vi "AddValue.vi"(1 "Display State In":T2 caption="State", 2 "Data In":T1) -> (0 "Display State Out":T2 caption="State")   [LabVIEW 2013, in "VariantXControl__VP.xctl"]
uses:
  VariantXControl__VP.xctl
  VariantState.ctl
  Permissions.ctl
  TreeSettings.ctl
  VariantData.ctl
  VariantTree__VP.lvclass
  Browse Variant_SetRef.vi
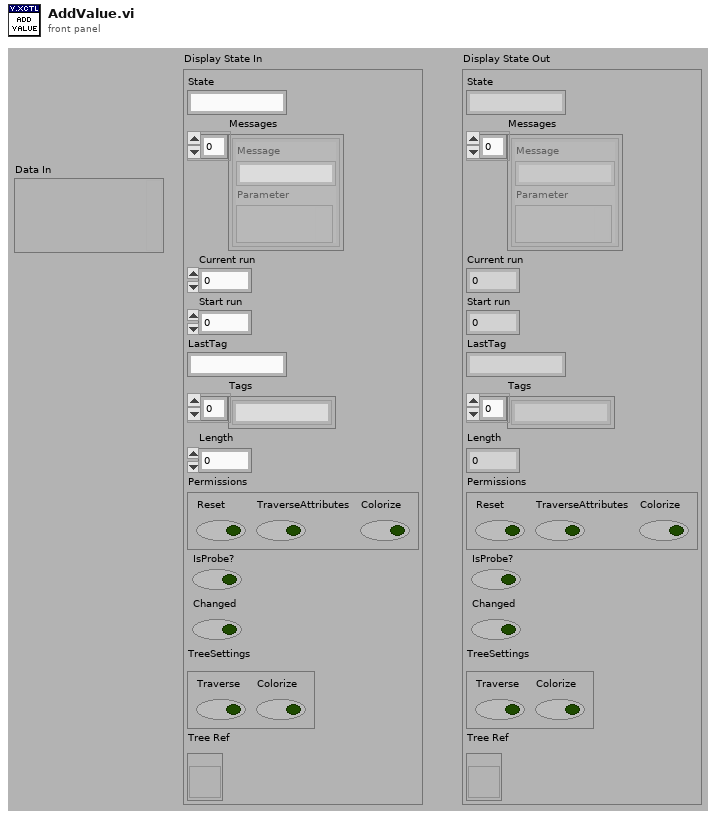
[diagram p1: front panel]
types:
  T1 = typedef "VariantXControl__VP.xctl/VariantData.ctl" = variant
  T2 = typedef "VariantXControl__VP.xctl/VariantState.ctl" = cluster{"State":string, "Messages":cluster{"Message":string, "Parameter":variant}[], "Current run":i32, "Start run":i32, "LastTag":string, "Tags":string[], "Length":i32, "Permissions":T3, "IsProbe?":bool, "Changed":bool, "TreeSettings":T4, "Tree Ref":refnum<vi>}
  T3 = typedef "VariantXControl__VP.xctl/Permissions.ctl" = cluster{"Reset":bool, "TraverseAttributes":bool, "Colorize":bool}
  T4 = typedef "VariantXControl__VP.xctl/TreeSettings.ctl" = cluster{"Traverse":bool, "Colorize":bool}
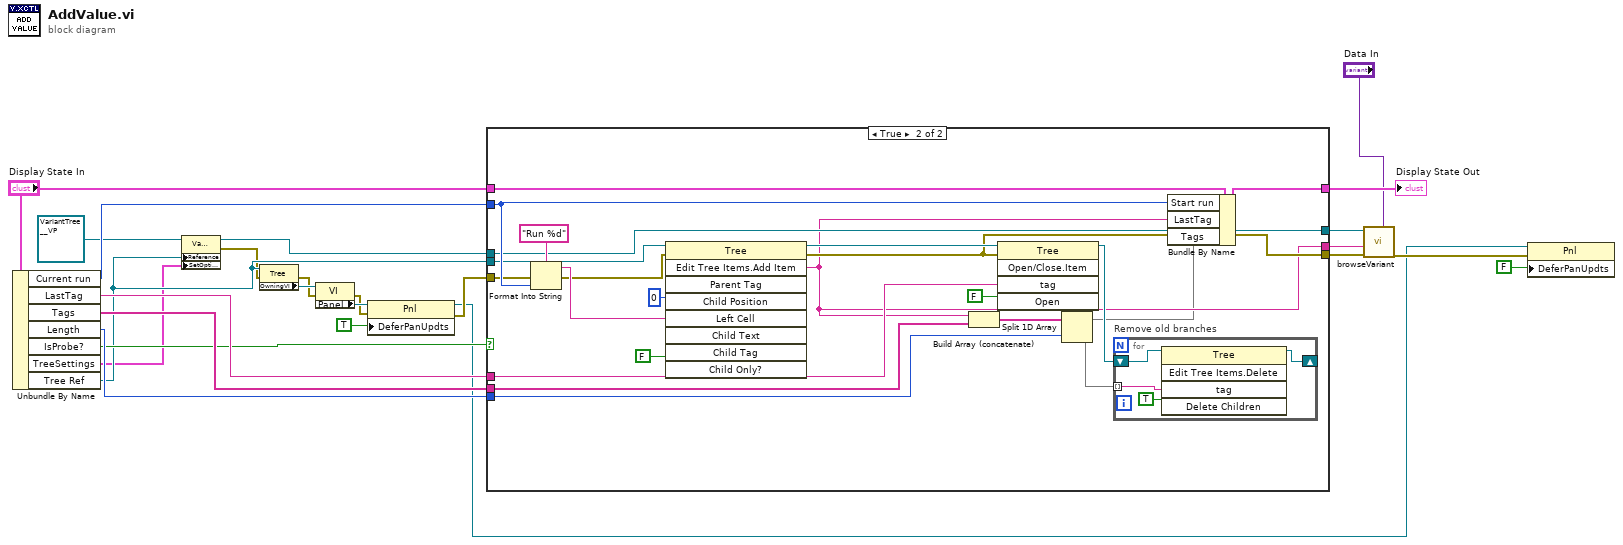
[diagram p0: block diagram]
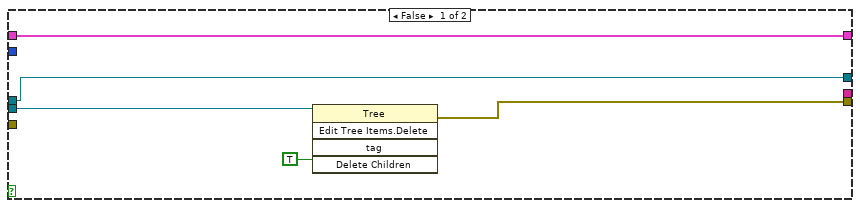
[diagram p2: hidden frame]
diagram:
  n1 = Unbundle By Name("Display State In") -> ("Current run"=w22:i32, "LastTag"=w19:string, "Tags"=w20:string[], "Length"=w21:i32, "IsProbe?"=w15:bool, "TreeSettings"=w3:T4, "Tree Ref"=w4:refnum<vi>)
  n2 = property class="VariantTree__VP.lvclass"(reference=refnum<class "VariantTree__VP.lvclass"> refnum ("Dummy Class.lvclass"), "Reference"=w4, "SetOptions"=w3) -> (reference out=w1:refnum<class "VariantTree__VP.lvclass">, error out=w2:errorcluster)  [unwired: 1 in]
  n3 = property class="Tree"(reference=w4, error in=w2) -> (error out=w13:errorcluster, "OwningVI"=w14:refnum<vi>)  [unwired: 1 out]
  n4 = property class="VI"(reference=w14, error in=w13) -> (error out=w10:errorcluster, "Panel"=w12:refnum<vi>)  [unwired: 1 out]
  n5 = property class="Pnl"(reference=w12, error in=w10, "DeferPanUpdts"=TRUE ("Defer Panel Updates")) -> (reference out=w6:refnum<vi>, error out=w9:errorcluster)
  n6 = case shown="True" w15 {
    tunnel: [w30 w52] -> w25
    tunnel: "Display State In" -> [w30 w51]
    tunnel: w22 -> [_ w50]
    tunnel: w21 -> [_ w47]
    tunnel: w20 -> [_ w45]
    tunnel: w19 -> [_ w44]
    tunnel: [_ w32] -> w18
    tunnel: w1 -> [w29 w35]
    tunnel: [w29 w35] -> w17
    tunnel: [w26 w33] -> w16
    tunnel: w4 -> [w27 w38]
    tunnel: w9 -> [_ w36]
    frame False {
      n7 = invoke class="Tree" method="Edit Tree Items.Delete"(reference=w27, "Delete Children"=TRUE ("Delete Children?")) -> (error out=w26:errorcluster)  [unwired: 3 in, 4 out]
    }
    frame True {
      n8 = Format Into String(format string="Run %d" ("Left Cell String"), error in=w36, w50) -> (resulting string=w42:string, error out=w37:errorcluster)  [unwired: 1 in]
      n9 = invoke class="Tree" method="Edit Tree Items.Add Item"(reference=w38, error in=w37, "Child Position"=0, "Left Cell"=w42, "Child Only?"=FALSE) -> (reference out=w34:refnum<vi>, error out=w33:errorcluster, "Edit Tree Items:Add Item"=w32:string)  [unwired: 4 in, 6 out]
      n10 = Build Array (concatenate)(w32, w45) -> (w49:string[])
      n11 = invoke class="Tree" method="Open/Close.Item"(reference=w34, error in=w33, "tag"=w44, "Open"=FALSE ("Open?")) -> (reference out=w43:refnum<vi>)  [unwired: 1 in, 4 out]
      n12 = Split 1D Array(array=w49, index=w47) -> (first subarray=w31:string[], second subarray=w48:string[])
      n13 = for "Remove old branches" {
        tunnel: w48 -> [w55] mode=indexing
        shift-right: [w53] -> _
        shift-left: w43 -> [w54]
        n14 = invoke class="Tree" method="Edit Tree Items.Delete"(reference=w54, "tag"=w55, "Delete Children"=TRUE ("Delete Children?")) -> (reference out=w53:refnum<vi>)  [unwired: 2 in, 4 out]
      }
      n15 = Bundle By Name(cluster=w51, "Start run"=w50, "LastTag"=w32, "Tags"=w31) -> (w52:T2)
    }
  }
  "Display State Out" <- w25
  n16 = call-dynamic "browseVariant.vi"("Variant"="Data In", "error in (no error)"=w16, "ParentTag"=w18, "VariantProbe.lvclass in"=w17) -> ("error out"=w7:errorcluster)  [unwired: 4 in, 1 out]
  n17 = property class="Pnl"(reference=w6, error in=w7, "DeferPanUpdts"=FALSE ("Defer Panel Updates")) -> ()  [unwired: 2 out]
